vi "ASAP_SubVI.vi"(6 "Use LUT":bool, 7 "Log file refnum":refnum<file>, 8 "error in":errorcluster, 9 "Configuration":T2={"Calibration data"={"T1"=[], "K1"=[], "T2"=[], "K2"=[], "Sensor LUT"=array1x8x2x17[272 elements]}, "Block size"=0, "Tasks"={"Analog Input"="", "Counters"=[], "Digital out"=""}, "Light enables"=[]}, 10 "ADC data":dbl[][](array[numeric])=[[0.4233890953707781, 0.059737563753272625, -0.34526321832859963, -0.4370842281402643, -0.1850326932502861, 0.11627349522930426, 0.3480982972524768, 0.14520556157669487, -0.01859340351497344, -0.04275678381581041, 0.0034736843764850063, 0.02845318126523978, -0.05997519222712916, -0.31180249886316935, -0.1913055722069559, 0.09030184950540061, 0.360436060764886], [0.6090161583111819, 0.023732520276295323, -0.5218643351088168, -0.6243751263951983, -0.2834785113270817, 0.15024627064329113, 0.4894786524267905, 0.24355543536140833, 0.052680574834113765, 0.0051379172996168666, -0.03373152132429563, -0.04606924715825583, -0.18644089055291246, -0.46828867250845085, -0.19741842890272493, 0.2275371695300576, 0.5495514119082466], [-0.3627056826684615, 0.03133358461652651, 0.3305597941044889, 0.369221317860794, 0.17977042772246973, -0.09143559265147504, -0.2909675650457234, -0.16731821192728233, -0.07733762070534453, -0.03201928179911879, 0.04986418022173536, 0.07868421992524977, 0.1690489172928197, 0.28346509297598055, 0.06458624334066014, -0.19497008575623961, -0.34731150756447954], [-0.6450181281783133, 0.10571201219829456, 0.611512527243948, 0.6368442793097259, 0.1730174762656655, -0.318779482110553, -0.5129030504438435, -0.1320972814398578, 0.06778669197162364, 0.05759326324280886, -0.031955272844838026, -0.06567198903643284, 0.19175611740982554, 0.49285514286049803, 0.23913881034792678, -0.2701966435703145, -0.6145497005316812], [0.4695717653663261, -0.13065707989874734, -0.48157056823484895, -0.4650882160743811, -0.10884602816301027, 0.2719754623206629, 0.3716696684050737, 0.08025243985520478, -0.05592662595057675, -0.03766807199567128, 0.027317022173162845, 0.04933610623551206, -0.17896784359433077, -0.3703707665898961, -0.16486986906943993, 0.2394908601602379, 0.47870908960882014], [0.668160939441404, -0.26571601376575427, -0.7523298763225447, -0.6841118364455508, -0.18660091297417802, 0.4193565147222573, 0.5509276134493617, 0.16146384928902122, -0.01142440045017552, -0.025378352764062116, -0.011488409406532252, -0.004927491337157158, -0.3586731126626958, -0.5398829220356592, -0.15688475099700663, 0.4466084441328689, 0.748461004808878], [-0.3118825101365961, 0.1851791900696957, 0.4070827491012809, 0.3491544481283409, 0.12969938150207558, -0.21727721323812305, -0.2918476889082694, -0.1374740339016221, -0.07074469855287382, -0.0026391711111129917, 0.06805873010744334, 0.08567720073080362, 0.2530927857458196, 0.2521806565553053, -0.009680156386373016, -0.29677638264989614, -0.4047596372992107], [-0.6122773710321248, 0.443872048993655, 0.8820654900364707, 0.6474378529873531, 0.013395073062435703, -0.6203265386424837, -0.5113668303400581, -0.011152362385570862, 0.1554790069238322, 0.035622185214427414, -0.09994878350250055, -0.1158550087471243, 0.43435067511840836, 0.58534866769129, 0.18177070962625866, -0.5484281507089904, -0.8615301809255184], [-0.06624806961243182, -0.05802291916164041, -0.042420736809552224, -0.03131518330175245, -0.031459203448991, -0.04258075919349681, -0.051510008186773336, -0.051558014901649865, -0.04872561872163144, -0.04810153142705679, -0.04982977316526523, -0.05176604399943352, -0.044020960648023424, -0.03389154370964889, -0.03109115196155207, -0.04093252863778666, -0.05603864161838519], [-0.022401936357063147, -0.022561958744878777, -0.022497949789757297, -0.022241913969207668, -0.022017882626142776, -0.022001880387349414, -0.022113896058894494, -0.02216190277526494, -0.022225911730419923, -0.022241913969207668, -0.022321925163140396, -0.022481947550975934, -0.02243394083462946, -0.022225911730419923, -0.021953873670966927, -0.021873862476988058, -0.022113896058894494], [-0.04461304346772397, -0.04464504794445658, -0.04464504794445658, -0.04464504794445658, -0.04462904570609038, -0.04462904570609038, -0.04462904570609038, -0.04461304346772397, -0.04461304346772397, -0.04462904570609038, -0.04459704122935736, -0.04461304346772397, -0.04464504794445658, -0.044565036752623535, -0.04461304346772397, -0.044565036752623535, -0.04458103899099055], [-0.044565036752623535, -0.044565036752623535, -0.044533032275888895, -0.044533032275888895, -0.04454903451425632, -0.044565036752623535, -0.04454903451425632, -0.04459704122935736, -0.04451703003752128, -0.044533032275888895, -0.044533032275888895, -0.044565036752623535, -0.04459704122935736, -0.04462904570609038, -0.04461304346772397, -0.04461304346772397, -0.04461304346772397]], 11 "timestamp":cluster{"t0":timestamp, "dt":dbl}) -> (0 "error out":errorcluster, 1 "XYZ out":T1(array[cluster]), 2 "Raw signal":dbl[](graph), 3 "Demodulator out":waveform(sgl)[](graph), 5 "Diagnostics":cluster{"Valid position":bool, "Message":string})   [LabVIEW 2014]
uses:
  <vilib>/Analysis/Matrix/Datatypes/RealMatrix.ctl
  <vilib>/Analysis/Matrix/NI_Matrix.lvlib
  initialization/configuration.ctl
  initialization/asap_calibration.ctl
panel:
  in  "Display channel":i32 min=0 max=7
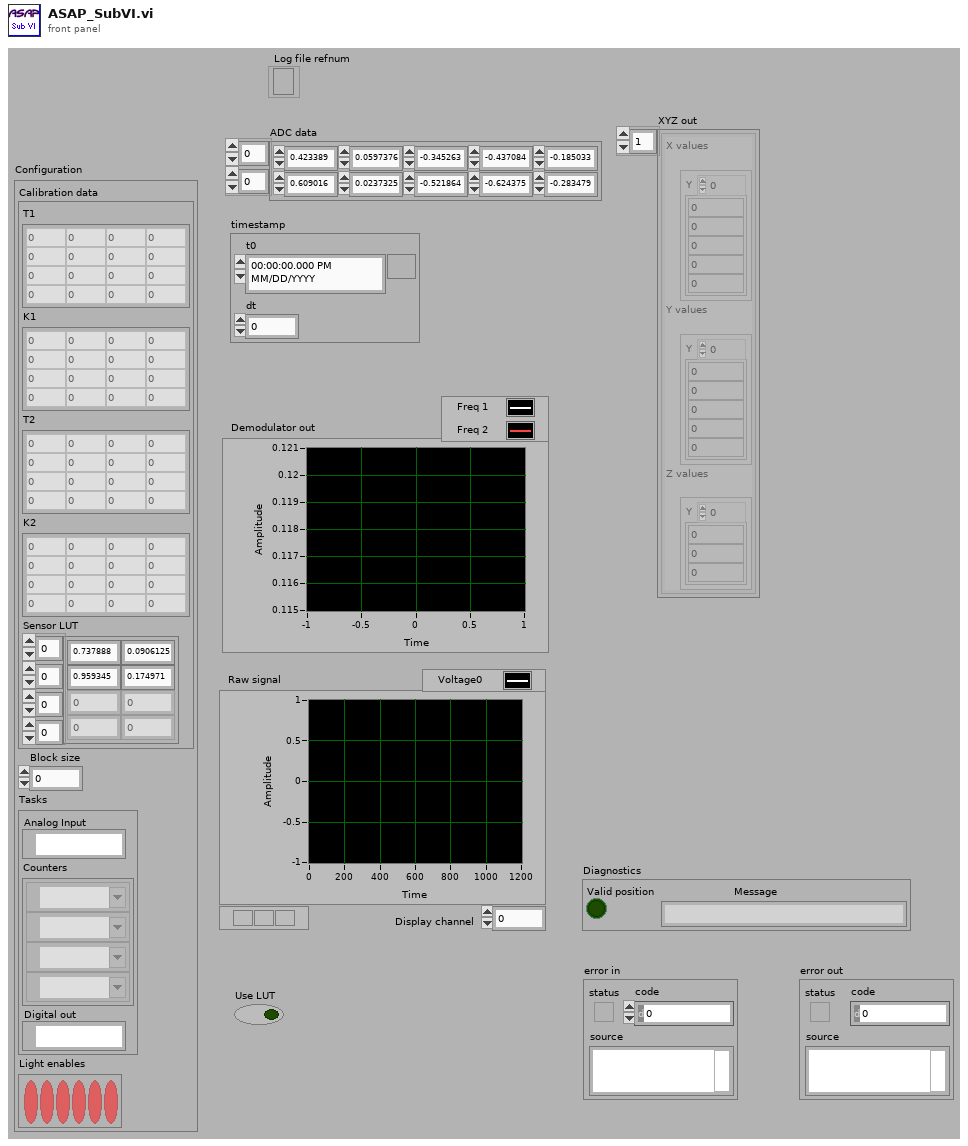
[diagram p1: front panel]
types:
  T1 = cluster{"X values":waveform(dbl), "Y values":waveform(dbl), "Z values":waveform(dbl)}[]
  T2 = typedef "configuration.ctl" = cluster{"Calibration data":T3, "Block size":i32, "Tasks":cluster{"Analog Input":refnum<k21>, "Counters":refnum<k21>[], "Digital out":refnum<k21>}, "Light enables":bool[]}
  T3 = typedef "asap_calibration.ctl" = cluster{"T1":T4, "K1":T4, "T2":T4, "K2":T4, "Sensor LUT":sgl[][][][]}
  T4 = typedef "NI_Matrix.lvlib/RealMatrix.ctl" = dbl[][]
  T5 = cluster{"X values":waveform(sgl), "Y values":waveform(sgl), "Z values":waveform(sgl)}[]
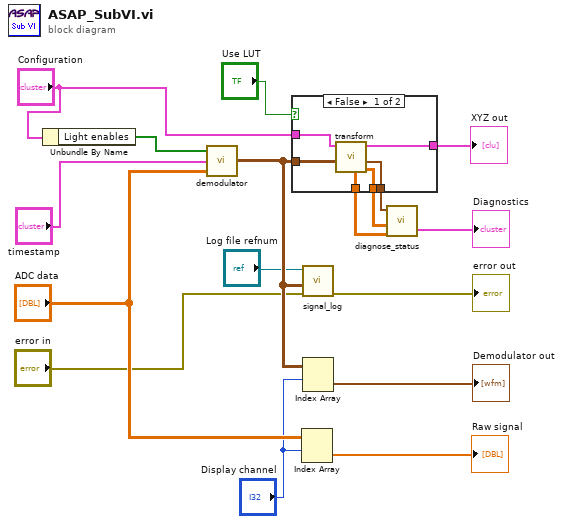
[diagram p0: block diagram]
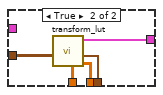
[diagram p2: hidden frame]
diagram:
  n1 = Unbundle By Name("Configuration") -> ("Light enables"=w2:bool[])
  n2 = call "demodulator.vi"("ADC data"="ADC data", "timestamp"="timestamp", "Demodulator table"=w2) -> ("Demodulated signals"=w14:waveform(sgl)[][])
  n3 = case shown="False" "Use LUT" {
    tunnel: w14 -> [w23 w28]
    tunnel: [w22 w26] -> w11
    tunnel: [w21 w24] -> w8
    tunnel: [w20 w25] -> w7
    tunnel: [w19 w27] -> w6
    tunnel: "Configuration" -> [w18 _]
    frame False {
      n4 = call "transform.vi"("Demodulated signals"=w23, "Configuration"=w18) -> ("Sum amplitudes"=w22:sgl[][], "Match error"=w20:waveform(sgl)[], "XYZ out"=w21:T5, "Axis positions"=w19:sgl[][])  [unwired: 6 out]
    }
    frame True {
      n5 = call "transform_lut.vi"("Demodulated signals"=w28) -> ("Sum amplitudes"=w26:sgl[][], "Match error"=w25:waveform(sgl)[], "XYZ out"=w24:T5, "Axis positions"=w27:sgl[][])  [unwired: 1 in, 6 out]
    }
  }
  "XYZ out" <- w8
  n6 = Index Array(array="ADC data", index (row)="Display channel") -> (element=→"Raw signal":dbl[])  [unwired: 1 in]
  n7 = call "signal_log.vi"("error in"="error in", "Demodulated signals"=w14, "Log file refnum"="Log file refnum") -> ("error out"=→"error out":errorcluster)  [unwired: 8 out]
  n8 = Index Array(array=w14, index (row)="Display channel") -> (element=→"Demodulator out":waveform(sgl)[])  [unwired: 1 in]
  n9 = call "diagnose_status.vi"("Match error"=w7, "Sum amplitudes"=w11, "Axis positions"=w6) -> ("Status"=→"Diagnostics":cluster{bool, string})  [unwired: 3 out]
